vi "Evaluate.vi"(0 "object in":refnum<class "Evaluator.lvclass">, 5 "error in (no error)":errorcluster) -> (14 "object out":refnum<class "Evaluator.lvclass">, 19 "error out":errorcluster)   [LabVIEW 2023]
uses:
  Evaluator.lvclass
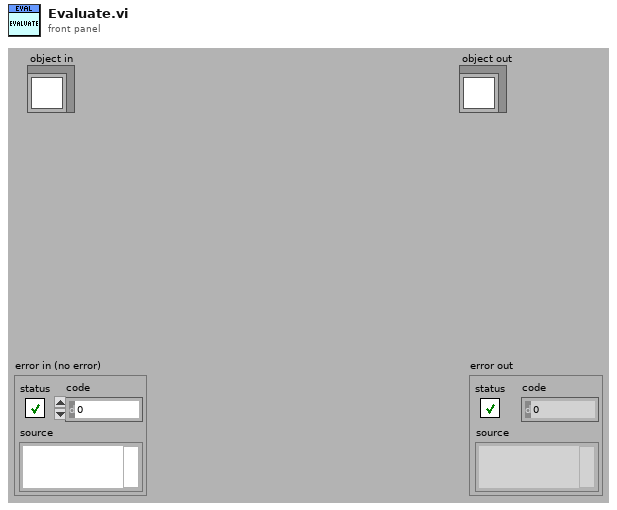
[diagram p1: front panel]
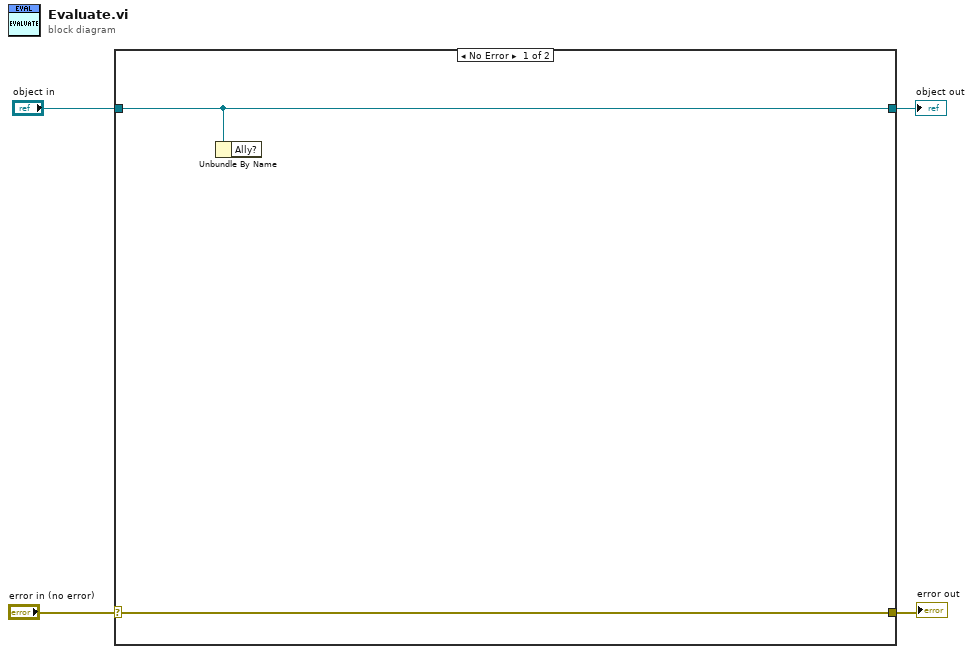
[diagram p0: block diagram]
diagram:
  n1 = case shown="No Error" "error in (no error)" {
    selector: "error in (no error)" -> [w6 w8]
    tunnel: [w6 w8] -> w3
    tunnel: [w5 w7] -> w1
    tunnel: "object in" -> [w5 w7]
    frame No Error {
      n2 = Unbundle By Name(w5) -> ()  [unwired: 1 out]
    }
    frame Error {
    }
  }
  "error out" <- w3
  "object out" <- w1
